vi "SetAttributeViReal64_ACP_SE_TOI.vi"(7 "AttributeValue":dbl, 8 "error in (no error)":errorcluster {"code" format="%.0x"}, 9 "AttributeID":u32(ring)=1150139 items=["SA_ACP_CARRIER_CPSD"=1150139, "SA_ACP_CARRIER_REFERENCE_FREQUENCY"=1150140, "SA_ACP_CARRIER_REFERENCE_LEVEL"=1150142, "SA_ACP_DISPLAY_WINDOWY_REFERENCE"=1150148, "SA_ACP_DISPLAY_WINDOWY_SCALE"=1150151, "SA_ACP_FREQUENCY_SPAN"=1150154, "SA_ACP_MARKER_POSITION"=1150240, "SA_ACP_MARKER_TRACE_POINTS_POSITION"=1150746, "SA_ACP_OFFSETFILTER_ALPHA"=1150165, "SA_ACP_SWEEPCOUPLING_CHANNEL_INTEGRATION_BANDWIDTH"=1150131, "SA_ACP_SWEEPCOUPLING_RESOLUTION_BANDWIDTH"=1150132, "SA_ACP_SWEEPCOUPLING_SWEEP_TIME"=1150168, "SA_ACP_SWEEPCOUPLING_VIDEO_BANDWIDTH"=1150136, "SA_SPURIOUSEMISSIONS_DISPLAY_WINDOWY_REFERENCE"=1150435, "SA_SPURIOUSEMISSIONS_DISPLAY_WINDOWY_SCALE"=1150436, "SA_SPURIOUSEMISSIONS_MARKER_POSITION"=1150445, "SA_SPURIOUSEMISSIONS_MARKER_TRACE_POINTS_POSITION"=1150752, "SA_THIRDORDERINTERCEPT_DISPLAYWINDOWY_REFERENCE"=1150579, "SA_THIRDORDERINTERCEPT_DISPLAYWINDOWY_SCALE"=1150581, "SA_THIRDORDERINTERCEPT_LOWER_TONE_FREQUENCY"=1150497, "SA_THIRDORDERINTERCEPT_MAX_MIXER_LEVEL"=1150501, "SA_THIRDORDERINTERCEPT_SPAN"=1150500, "SA_THIRDORDERINTERCEPT_SWEEPCOUPLING_BANDWIDTH_RATIO"=1150493, "SA_THIRDORDERINTERCEPT_SWEEPCOUPLING_RESOLUTION_BANDWIDTH"=1150486, "SA_THIRDORDERINTERCEPT_SWEEPCOUPLING_SPAN_TO_RESOLUTION_BANDWIDTH_RATIO"=1150503, "SA_THIRDORDERINTERCEPT_SWEEPCOUPLING_SWEEP_TIME"=1150489, "SA_THIRDORDERINTERCEPT_SWEEPCOUPLING_VIDEO_BANDWIDTH"=1150491, "SA_THIRDORDERINTERCEPT_UPPER_TONE_FREQUENCY"=1150496, "SA_THIRDORDERINTERCEPT_ZEROSPANSWEEPCOUPLING_RESOLUTION_BANDWIDTH"=1150505, "SA_THIRDORDERINTERCEPT_ZEROSPANSWEEPCOUPLING_SWEEP_TIME"=1150508], 11 "instrument handle":refnum<k15>) -> (0 "error out":errorcluster {"code" format="%.0x"}, 3 "instrument handle out":refnum<k15>)   [LabVIEW 2009, in "Keysight XSAn.lvlib"]
doc: "Sets a Real64 attribute from the instrument driver.\nThe following Attributes are supported:\n\nSA_ACP_CARRIER_CPSD\nSA_ACP_CARRIER_REFERENCE_FREQUENCY\nSA_ACP_CARRIER_REFERENCE_LEVEL\nSA_ACP_DISPLAY_WINDOWY_REFERENCE\nSA_ACP_DISPLAY_WINDOWY_SCALE\nSA_ACP_FREQUENCY_SPAN\nSA_ACP_MARKER_POSITION\nSA_ACP_MARKER_TRACE_POINTS_POSITION\nSA_ACP_OFFSETFILTER_ALPHA\nSA_ACP_SWEEPCOUPLING_CHANNEL_INTEGRATION_BANDWIDTH\nSA_ACP_SWEEPCOUPLING_RESOLUTION_BANDWIDTH\nSA_ACP_SWEEPCOUPLING_SWEEP_TIME\nSA_ACP_SWEEPCOUPLING_VIDEO_BANDWIDTH\nSA_SPURIOUSEMISSIONS_DISPLAY_WINDOWY_REFERENCE\nSA_SPURIOUSEMISSIONS_DISPLAY_WINDOWY_SCALE\nSA_SPURIOUSEMISSIONS_MARKER_POSITION\nSA_SPURIOUSEMISSIONS_MARKER_TRACE_POINTS_POSITION\nSA_THIRDORDERINTERCEPT_DISPLAYWINDOWY_REFERENCE\nSA_THIRDORDERINTERCEPT_DISPLAYWINDOWY_SCALE\nSA_THIRDORDERINTERCEPT_LOWER_TONE_FREQUENCY\nSA_THIRDORDERINTERCEPT_MAX_MIXER_LEVEL\nSA_THIRDORDERINTERCEPT_SPAN\nSA_THIRDORDERINTERCEPT_SWEEPCOUPLING_BANDWIDTH_RATIO\nSA_THIRDORDERINTERCEPT_SWEEPCOUPLING_RESOLUTION_BANDWIDTH\nSA_THIRDORDERINTERCEPT_SWEEPCOUPLING_SPAN_TO_RESOLUTION_BANDWIDTH_RATIO\nSA_THIRDORDERINTERCEPT_SWEEPCOUPLING_SWEEP_TIME\nSA_THIRDORDERINTERCEPT_SWEEPCOUPLING_VIDEO_BANDWIDTH\nSA_THIRDORDERINTERCEPT_UPPER_TONE_FREQUENCY\nSA_THIRDORDERINTERCEPT_ZEROSPANSWEEPCOUPLING_RESOLUTION_BANDWIDTH\nSA_THIRDORDERINTERCEPT_ZEROSPANSWEEPCOUPLING_SWEEP_TIME"
uses:
  <instrlib>/Keysight XSAn/Keysight XSAn.lvlib
  AgXSAn.dll
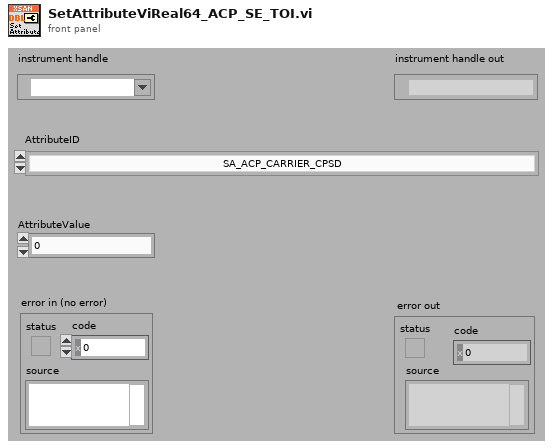
[diagram p1: front panel]
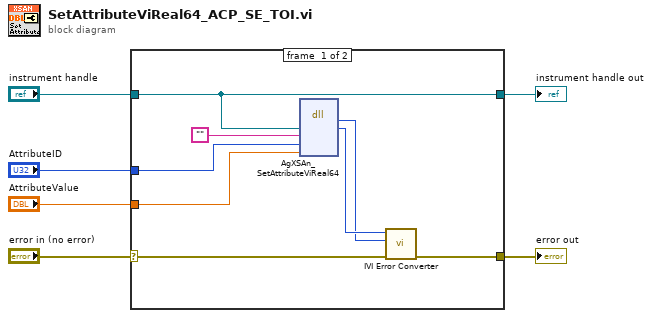
[diagram p0: block diagram]
diagram:
  n1 = case shown="No Error" "error in (no error)" {
    selector: "error in (no error)" -> [w12 w16]
    tunnel: [w11 w16] -> w6
    tunnel: "instrument handle" -> [w8 w15]
    tunnel: "AttributeID" -> [w10 _]
    tunnel: "AttributeValue" -> [w9 _]
    tunnel: [w8 w15] -> w1
    frame #0 {
      n2 = dll-call lib="AgXSAn**.dll" fn="AgXSAn_SetAttributeViReal64"("Vi"=w8, "RepCapIdentifier"="", "AttributeID"=w10, "AttributeValue"=w9) -> ("return type"=w13:i32, "Vi"=w14:u32)  [unwired: 6 in, 2 out]
      n3 = call <instrlib>:"IVI Error Converter.vi"("error in (no error)"=w12, "IVI error code (0)"=w13, "instrument handle"=w14) -> ("error out"=w11:errorcluster)  [unwired: 7 in, 1 out]
    }
    frame #1 {
    }
  }
  "error out" <- w6
  "instrument handle out" <- w1
